vi "GEECS tcp read single variable.vi"(8 "error in (no error)":errorcluster, 9 "timeout ms (2000)":i32=2000, 10 "clear buffer after read":bool, 11 "TCP Network Connection in":refnum<k5>) -> (0 "error out":errorcluster, 1 "timed out":bool, 2 "variable value":string, 3 "TCP Network Connection out":refnum<k5>)   [LabVIEW 2020]
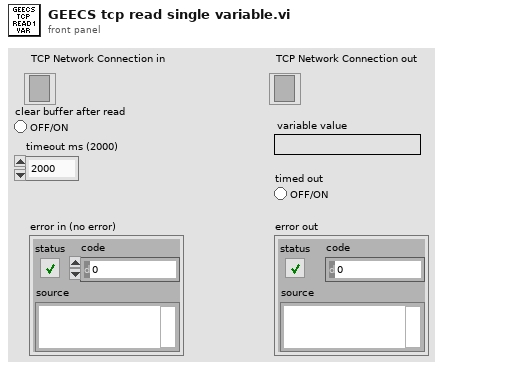
[diagram p1: front panel]
types:
  T1 = enum16{"Standard", "Buffered", "CRLF", "Immediate"}
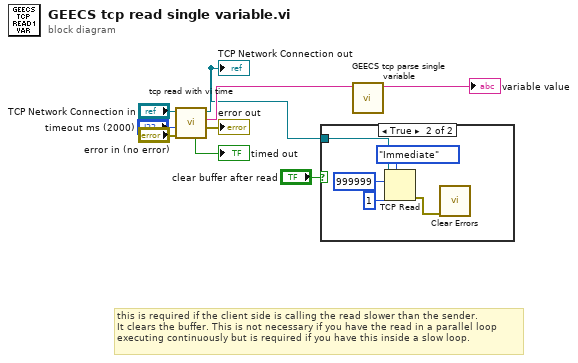
[diagram p0: block diagram]
diagram:
  # "this is required if the client side is calling the read slower than the sender. \nIt clears the buffer. This is not necessary if you have the read in a parallel loop\nexecuting continuously but is required if you have this inside a slow loop."
  n1 = call "tcp read with vi time.vi"("error in"="error in (no error)", "timeout ms (2000)"="timeout ms (2000)", "TCP Network Connection in"="TCP Network Connection in") -> ("error out"=→"error out":errorcluster, "data out"=w8:string, "TCP Network Connection out"=w3:refnum<k5>, "timed out"=→"timed out":bool)  [unwired: 4 in, 1 out]
  "TCP Network Connection out" <- w3
  n2 = case shown="True" "clear buffer after read" {
    tunnel: w3 -> [_ w14]
    frame False {
    }
    frame True {
      n3 = TCP Read(connection ID=w14, bytes to read=999999, 7:T1."Immediate" ("mode (standard)"), 9:1 ("timeout ms (25000)")) -> (error out=w10:errorcluster)  [unwired: 1 in, 2 out]
      n4 = call <vilib>:"Clear Errors.vi"("error in (no error)"=w10) -> ()  [unwired: 5 in, 2 out]
    }
  }
  n5 = call "GEECS tcp parse single variable.vi"("data in"=w8) -> ("variable value"=→"variable value":string)  [unwired: 10 in]
